vi "time_measure.vi"() -> ()   [LabVIEW 2020]
uses:
  <vilib>/Analysis/baseanly.llb/Mean (DBL).vi
  <vilib>/Analysis/NI_AALBase.lvlib
panel:
  out "error":i32
  out "x-y":dbl
  out "output array":u32[](array[numeric])
  out "counts":i32
  out "mean change time":dbl format="%0.2f"
  in  "Boolean":bool=TRUE
  out "mean measure time":dbl format="%0.2f"
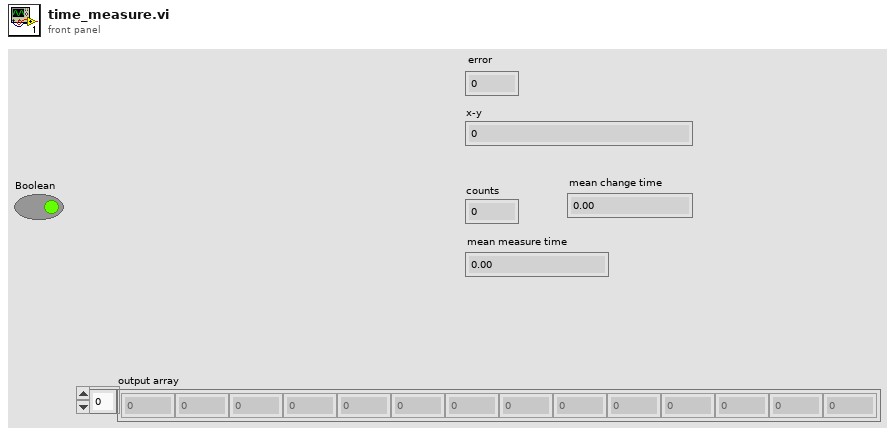
[diagram p1: front panel]
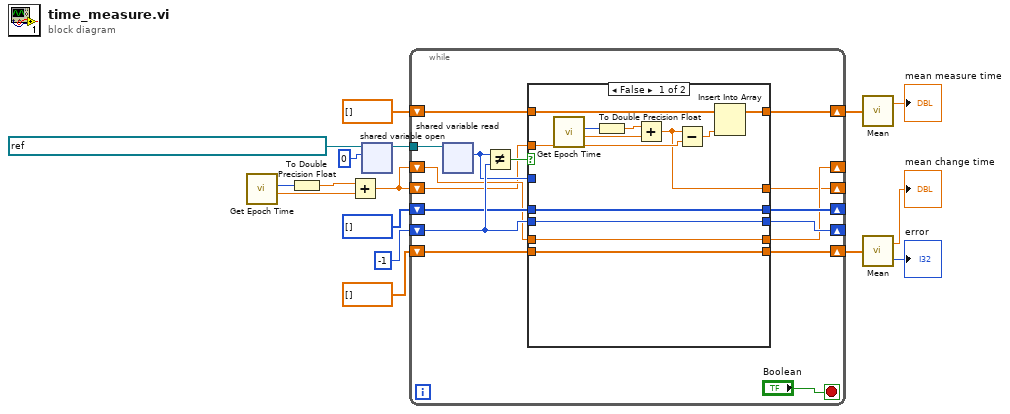
[diagram p0: block diagram]
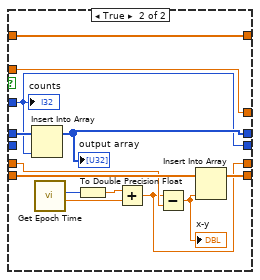
[diagram p2: hidden frame]
diagram:
  n1 = call <vilib>:"Get Epoch Time.vi"() -> ("Fractional Second"=w7:dbl, "Epoch Time (s)"=w6:i64)  [unwired: 9 in, 1 out]
  n2 = To Double Precision Float(number=w6) -> (double precision float=w5:dbl)
  n3 = Add(x=w5, y=w7) -> (x+y=w1:dbl)
  n4 = shared-variable-open(refnum<k21> "ni.var.psp://my computer/elyse_variables/elyse_counts" ("shared variable refnum in"), 0) -> (w14:refnum<k21>)  [unwired: 2 in, 1 out]
  n5 = while {
    tunnel: w14 -> [w31]
    shift-right: [w29] -> _
    shift-left: -1 -> [w30]
    shift-right: [w27] -> w9
    shift-left: ext[] [] -> [w28]
    shift-right: [w25] -> _
    shift-left: u32[] [] -> [w26]
    shift-right: [w21] -> _
    shift-left: w1 -> [w22]
    shift-right: [w19] -> w2
    shift-left: ext[] [] -> [w20]
    shift-right: [w17] -> _
    shift-left: w1 -> [w18]
    stop <- "Boolean" stop-if-true
    n6 = shared-variable-read(w31) -> (w23:i32)  [unwired: 1 in, 3 out]
    n7 = Not Equal?(x=w23, y=w30) -> (x != y?=w24:bool)
    n8 = case shown="False" w24 {
      tunnel: w30 -> [w44 _]
      tunnel: [w44 w53] -> w29
      tunnel: w28 -> [w43 w57]
      tunnel: [w43 w56] -> w27
      tunnel: w26 -> [w42 w55]
      tunnel: [w42 w54] -> w25
      tunnel: w23 -> [_ w53]
      tunnel: w22 -> [w41 w49]
      tunnel: [w41 w47] -> w21
      tunnel: w20 -> [w37 w46]
      tunnel: [w36 w46] -> w19
      tunnel: w18 -> [w35 w45]
      tunnel: [w33 w45] -> w17
      frame False {
        n9 = call <vilib>:"Get Epoch Time.vi"() -> ("Fractional Second"=w38:dbl, "Epoch Time (s)"=w40:i64)  [unwired: 9 in, 1 out]
        n10 = To Double Precision Float(number=w40) -> (double precision float=w39:dbl)
        n11 = Add(x=w39, y=w38) -> (x+y=w33:dbl)
        n12 = Subtract(x=w33, y=w35) -> (x-y=w34:dbl)
        n13 = Insert Into Array(array=w37, new element=w34) -> (w36:ext[])  [unwired: 1 in]
      }
      frame True {
        n14 = Insert Into Array(array=w55, new element=w53) -> (w54:u32[])  [unwired: 1 in]
        "output array" <- w54
        n15 = call <vilib>:"Get Epoch Time.vi"() -> ("Fractional Second"=w50:dbl, "Epoch Time (s)"=w52:i64)  [unwired: 9 in, 1 out]
        n16 = To Double Precision Float(number=w52) -> (double precision float=w51:dbl)
        n17 = Add(x=w51, y=w50) -> (x+y=w47:dbl)
        n18 = Subtract(x=w47, y=w49) -> (x-y=w48:dbl)
        "x-y" <- w48
        n19 = Insert Into Array(array=w57, new element=w48) -> (w56:ext[])  [unwired: 1 in]
        "counts" <- w53
      }
    }
  }
  n20 = call-poly <vilib>:"Mean.vi"("X"=w2) -> ("mean"=→"mean measure time":dbl)  [unwired: 1 out]
  n21 = call-poly <vilib>:"Mean.vi"("X"=w9) -> ("mean"=→"mean change time":dbl, "error"=→"error":i32)
